vi "test_axsun_stephan.vi"() -> ()   [LabVIEW 2018]
uses:
  cluster_Axsun.ctl
  Action_Axsun.ctl
panel:
  out "Initialization error":errorcluster
  in  "stop":bool
  out "output cluster":T1
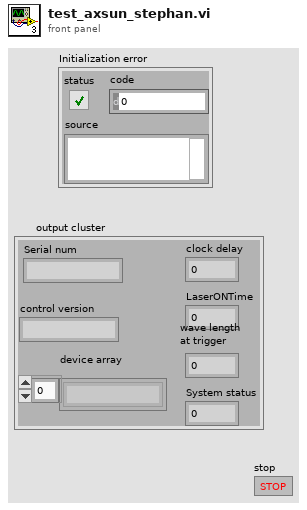
[diagram p1: front panel]
types:
  T1 = typedef "cluster_Axsun.ctl" = cluster{"device array":string[], "control version":string, "Serial num":string, "LaserONTime":i32, "wave length\nat trigger":dbl, "System status":dbl, "clock delay":u32}
  T2 = typedef "Action_Axsun.ctl" = enum16{"Init", "Stop", "Source current ON", "Source current OFF", "Laser ON", "Laser OFF", "GetLaserOnTime", "Clock delay"}
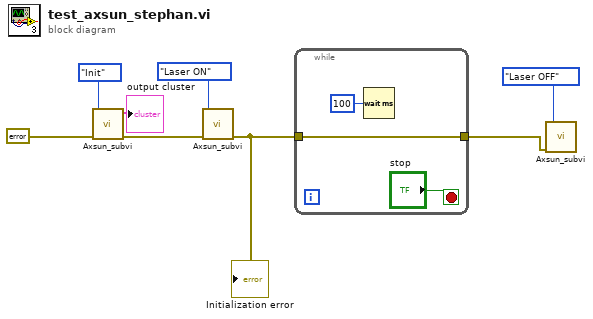
[diagram p0: block diagram]
diagram:
  n1 = call "Axsun_subvi.vi"("error in (no error)"=errorcluster {"status"=FALSE, "code"=0, "source"=""}, "Action"=Action_Axsun."Init") -> ("error out"=w5:errorcluster, "output cluster"=→"output cluster":T1)  [unwired: 8 in]
  n2 = call "Axsun_subvi.vi"("error in (no error)"=w5, "Action"=Action_Axsun."Laser ON") -> ("error out"=w1:errorcluster)  [unwired: 8 in, 1 out]
  "Initialization error" <- w1
  n3 = while {
    tunnel: [w11] -> w2
    tunnel: w1 -> [w11]
    stop <- "stop" stop-if-true
    n4 = Wait (ms)(milliseconds to wait=u32 100) -> ()  [unwired: 1 out]
  }
  n5 = call "Axsun_subvi.vi"("error in (no error)"=w2, "Action"=Action_Axsun."Laser OFF") -> ()  [unwired: 8 in, 2 out]
